vi "Init SharedVariables.vi"(11 "Boolean in":refnum<vi>) -> (0 "error out":errorcluster)   [LabVIEW 2018]
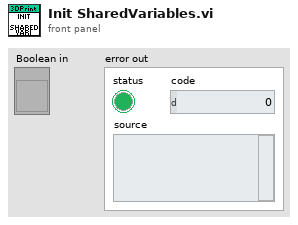
[diagram p1: front panel]
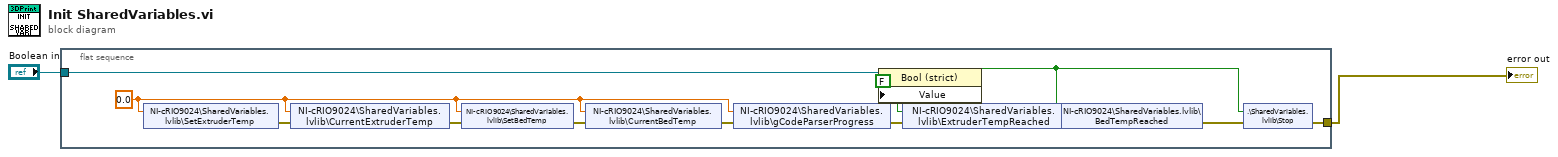
[diagram p0: block diagram]
diagram:
  n1 = flat-sequence {
    tunnel: [w7] -> w2
    tunnel: "Boolean in" -> [w3]
    frame #0 {
      w4 = 0.0 ("Set Extruder Temp")
      w6 = FALSE ("Stop")
      n2 = shared-variable "NI-cRIO9024\\SharedVariables.lvlib\\SetExtruderTemp"(w4) -> (error out=w5:errorcluster)  [unwired: 1 in]
      n3 = shared-variable "NI-cRIO9024\\SharedVariables.lvlib\\CurrentExtruderTemp"(w4, error in=w5) -> (error out=w13:errorcluster)
      n4 = shared-variable "NI-cRIO9024\\SharedVariables.lvlib\\SetBedTemp"(w4, error in=w13) -> (error out=w12:errorcluster)
      n5 = shared-variable "NI-cRIO9024\\SharedVariables.lvlib\\CurrentBedTemp"(w4, error in=w12) -> (error out=w11:errorcluster)
      n6 = shared-variable "NI-cRIO9024\\SharedVariables.lvlib\\gCodeParserProgress"(w4, error in=w11) -> (error out=w10:errorcluster)
      n7 = property class="Bool (strict)"(reference=w3, "Value"=w6) -> ()  [unwired: 1 in, 2 out]
      n8 = shared-variable "NI-cRIO9024\\SharedVariables.lvlib\\ExtruderTempReached"(w6, error in=w10) -> (error out=w9:errorcluster)
      n9 = shared-variable "NI-cRIO9024\\SharedVariables.lvlib\\BedTempReached"(w6, error in=w9) -> (error out=w8:errorcluster)
      n10 = shared-variable ".\\SharedVariables.lvlib\\Stop"(w6, error in=w8) -> (error out=w7:errorcluster)
    }
  }
  "error out" <- w2
